vi "AMI_Parse_Desimanar_Y.vi"(8 "error in (no error)":errorcluster, 11 "String":string="Axis Y demagnetize in 15 steps at 0.030Tesla/min, waiting 10 sec") -> (0 "error out":errorcluster, 1 "Y Wait secs":i32, 2 "Y Rate":dbl, 3 "Y Steps":i32)   [LabVIEW 2017]
panel:
  # "Axis Y demagnetize in 15 steps at 0.030Tesla/min, waiting 10 sec"
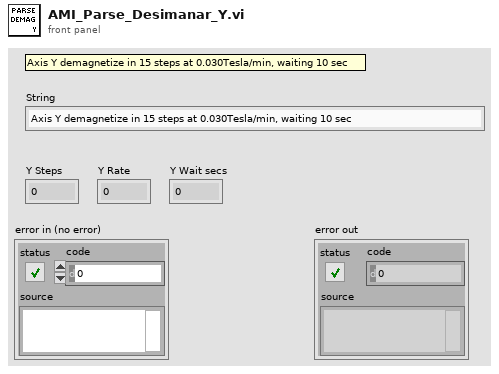
[diagram p1: front panel]
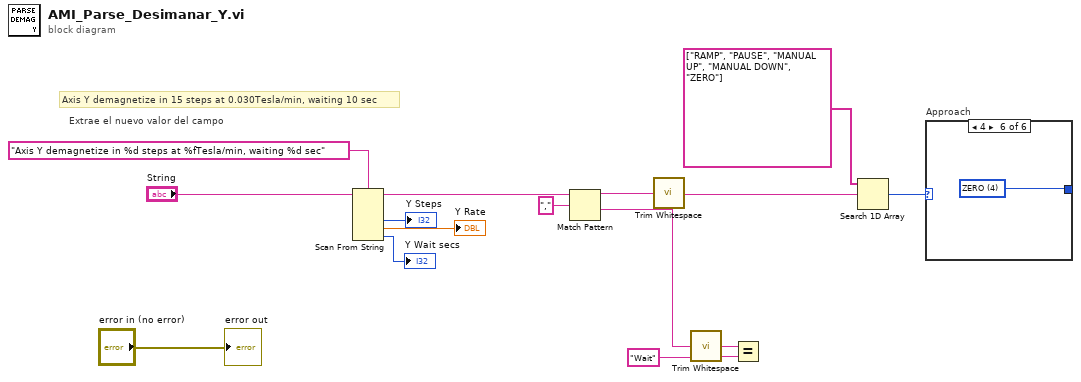
[diagram p0: block diagram]
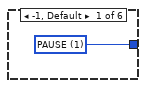
[diagram p2: hidden frame]
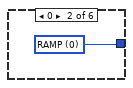
[diagram p3: hidden frame]
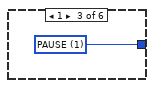
[diagram p4: hidden frame]
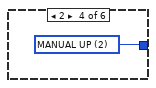
[diagram p5: hidden frame]
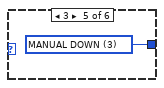
[diagram p6: hidden frame]
diagram:
  # "Axis Y demagnetize in 15 steps at 0.030Tesla/min, waiting 10 sec"
  # "Extrae el nuevo valor del campo"
  n1 = Scan From String(format string="Axis Y demagnetize in %d steps at %fTesla/min, waiting %d sec", input string="String") -> (remaining string=w5:string, output 1=→"Y Steps":i32, output 2=→"Y Rate":dbl, output 3=→"Y Wait secs":i32)  [unwired: 5 in, 2 out]
  n2 = Match Pattern(string=w5, regular expression=",") -> (before substring=w7:string, after substring=w4:string)  [unwired: 1 in, 2 out]
  n3 = call <vilib>:"Trim Whitespace.vi"("string"=w7) -> ("trimmed string"=w3:string)  [unwired: 1 in]
  n4 = call <vilib>:"Trim Whitespace.vi"("string"=w4) -> ("trimmed string"=w6:string)  [unwired: 1 in]
  n5 = Equal?(x=w6, y="Wait" ("after substring")) -> ()  [unwired: 1 out]
  n6 = Search 1D Array(1D array=string[] ["RAMP", "PAUSE", "MANUAL UP", "MANUAL DOWN", "ZERO"], element=w3) -> (index of element=w11:i32)  [unwired: 1 in]
  n7 = case "Approach" shown="4" w11 {
    tunnel: [w16 w17 w18 w19 w20 w21] -> _
    frame -1, Default {
      w16 = u16 1 items=["RAMP", "PAUSE", "MANUAL UP", "MANUAL DOWN", "ZERO"] ("Modo Rampa")
    }
    frame 0 {
      w17 = u16 0 items=["RAMP", "PAUSE", "MANUAL UP", "MANUAL DOWN", "ZERO"] ("Modo Rampa")
    }
    frame 1 {
      w18 = u16 1 items=["RAMP", "PAUSE", "MANUAL UP", "MANUAL DOWN", "ZERO"] ("Modo Rampa")
    }
    frame 2 {
      w19 = u16 2 items=["RAMP", "PAUSE", "MANUAL UP", "MANUAL DOWN", "ZERO"] ("Modo Rampa")
    }
    frame 3 {
      w20 = u16 3 items=["RAMP", "PAUSE", "MANUAL UP", "MANUAL DOWN", "ZERO"] ("Modo Rampa")
    }
    frame 4 {
      w21 = u16 4 items=["RAMP", "PAUSE", "MANUAL UP", "MANUAL DOWN", "ZERO"] ("Modo Rampa")
    }
  }
  "error out" <- "error in (no error)"
